vi "OCT Differential.vi"() -> ()   [LabVIEW 2014]
doc: "I. Description:\nThis example demonstrates how to acquire a continuous amount of data (Waveform) using the DAQ device's internal clock.\n\nII. Instructions for Running:\n1. Create an analog input voltage channel.\n2. Set the rate for the sample clock. Additionally, define the sample mode to be continuous.\n3. Call the Start VI to start the acquisition.\n4. Read the waveform data in a loop until the user hits the stop button or an error occurs.\nNote: This example reads data from one or more channels and returns an array of data. Use the Index Array function to access an individual channel of data.\n5. Call the Clear Task VI to clear the Task.\n6. Use the popup dialog box to display an error if any.\n\nIV. I/O Connections Overview:\nMake sure your signal input terminal matches the Physical Channel I/O Control. For further connection information, refer to your hardware reference manual."
uses:
  ATS-VI/ATS_ctl/Device_Ctrl.ctl
  ATS-VI/ATS_ctl/ATS_Async_Ctrl.ctl
  ATS-VI/ATS_ctl/ATS_Async_Mode.ctl
  ATS-VI/ATS_ctl/ATS_DMA_Channel.ctl
  ATS-VI/ATS_ctl/ATS_ReadSamples.ctl
  ATS-VI/ATS_ctl/ATS_Check_Ctrl.ctl
  ATS-VI/ATS_ctl/ClockSource.ctl
  Galvo VIs/galvo_states.ctl
  Signal Processing/processing_states.ctl
  En Face/En Face States.ctl
  Saving Data/Saving Data States.ctl
  Type Defs/OCT Hardware States.ctl
  ATS-VI/ATS_ctl/Range.ctl
  ATS-VI/ATS_ctl/Impedance.ctl
  Type Defs/OCT Imaging Parameters Cluster.ctl
  Classes/Galvo/Scanning Cluster.ctl
  Classes/Galvo/Galvo.lvclass
  Type Defs/OCT DAQ Channel Data Type.ctl
  Type Defs/Display States.ctl
  ATS-VI/ATS_ctl/Coupling.ctl
  ATS-VI/ATS_ctl/Bandwidth.ctl
  ATS-VI/ATS_ctl/InputCtrl.ctl
  ATS-VI/ATS_ctl/TriggerEngine.ctl
  ATS-VI/ATS_ctl/ExtTrigRange.ctl
  ATS-VI/ATS_ctl/ExtTrigger.ctl
  ATS-VI/ATS_ctl/TriggerOperation.ctl
  ATS-VI/ATS_ctl/Trigger.ctl
  ATS-VI/ATS_ctl/ClockRate.ctl
  ATS-VI/ATS_ctl/ClockEdge.ctl
  ATS-VI/ATS_ctl/Clock.ctl
  ATS-VI/ATS_ctl/Record.ctl
  ATS-VI/ATS_ctl/ATS_Global.ctl
  ATS-VI/ATS_ctl/ATS_Async_Status.ctl
  En Face/En Face Depth Parameters.ctl
  ATS-VI/ATS_ctl/ATS_Async_Setting.ctl
panel:
  out "size(s)":i32
  out "First Time?":bool
  out "Save Data":bool
  in  "Async_Setting":T1
  out "Processing Finished":bool
  in  "Imaging Parameters":T2={"Points Per A-Scan"=0, "A-Scans per B-Scan"=0, "Voltage Range"=4.0, "Card Resolution (bits)"=16}
  in  "OCT Hardware States":T3=enum."Save Sweep"
  out "Save State":T4=enum."Initialize"
  out "Clock Length":u32=6304
  out "Reset DAQ":bool
  in  "Tab Control":T5(tab)
  in  "B-Scans Per Buffer":i32=4
  out "Async_Status":T6
  out "Current State":T3=enum."Set Resampling Array"
  in  "Channels":tag="Dev1/ao0:1"
  in  "Trigger Source":tag="/Dev1/PFI7"
  in  "Setup_In":T7={"Record"={"Count"=1, "Presize"=0, "Length"=640}, "Clock"={"ClckSource"=enum."External", "ClckRate"=18, "ClckEdge"=0, "Decimation"=0}, "Input A"={"Coupling"=enum."AC", "Range"=11, "Impedance"=enum."50 ohms", "Bandwidth"=enum."Full Bandwidth"}, "Input B"={"Coupling"=enum."AC", "Range"=4, "Impedance"=enum."50 ohms", "Bandwidth"=enum."Full Bandwidth"}, "Trigger"={"TrigOperation"=enum."Only X", "Timeout (s)"=1.0, "Trig. Delay"=0, "Engine X"={"Source"=enum."External", "Slope"=enum."Positive", "Level"=180}, "Engine Y"={"Source"=enum."Disable", "Slope"=enum."Positive", "Level"=128}, "ExtTrigControl"={"Coupling"=enum."DC", "Range"=enum."5 V"}}} {"Clock"."ClckEdge" items=["Rising", "Falling"]; "Clock"."ClckRate" items=["1 kS/s", "2 kS/s", "5 kS/s", "10 kS/s", "20 kS/s", "50 kS/s", "100 kS/s", "200 kS/s", "500 kS/s", "1 MS/s", "2 MS/s", "5 MS/s", "10 MS/s", "20 MS/s", "25 MS/s", "50 MS/s", "100 MS/s", "125 MS/s", "200 MS/s", "250 MS/s", "500 MS/s", "1 GS/s"]; "Input B"."Range" items=["20mv", "40mV", "50mV", "80mV", "100mV", "200mV", "400mV", "500mV", "800mV", "1 V", "2 V", "4 V", "5 V", "8 V", "10 V", "20 V"]; "Trigger"."Timeout (s)" format="%.2f"; "Input A"."Range" items=["20mv", "40mV", "50mV", "80mV", "100mV", "200mV", "400mV", "500mV", "800mV", "1 V", "2 V", "4 V", "5 V", "8 V", "10 V", "20 V"]}
  in  "Data Format":T23
  out "Channel A or B Phase (or Channel B Raw)":sgl[][](graph)
  out "Channel A or B Intensity (or Channel A Raw)":sgl[][](graph)
  in  "Display":T24
  out "En Face":dbl[][](graph)
  in  "En Face Parameters":T25={"En Face Start\nDepth"=50, "En Face End\nDepth"=200}
  in  "Save Sweep":bool
  in  "Scanning":T26={"Fast Axis Offset"=300.0, "Slow Axis Offset"=1.0, "Slow Axis Amp"=8.0, "Fast Axis Amp"=8.0, "B-scans (rings)"=1, "A(cluster)/B"=0, "Scan Pattern"=enum."Raster"} {"A(cluster)/B" max=1000 step=1; "B-scans (rings)" max=1000 step=1; "Fast Axis Amp" max=20 format="%#.2f"; "Slow Axis Amp" max=20 format="%#.2f"; "Slow Axis Offset" max=10 format="%#.2f"; "Fast Axis Offset" max=10 format="%#.2f"}
  in  "Stop Button":bool
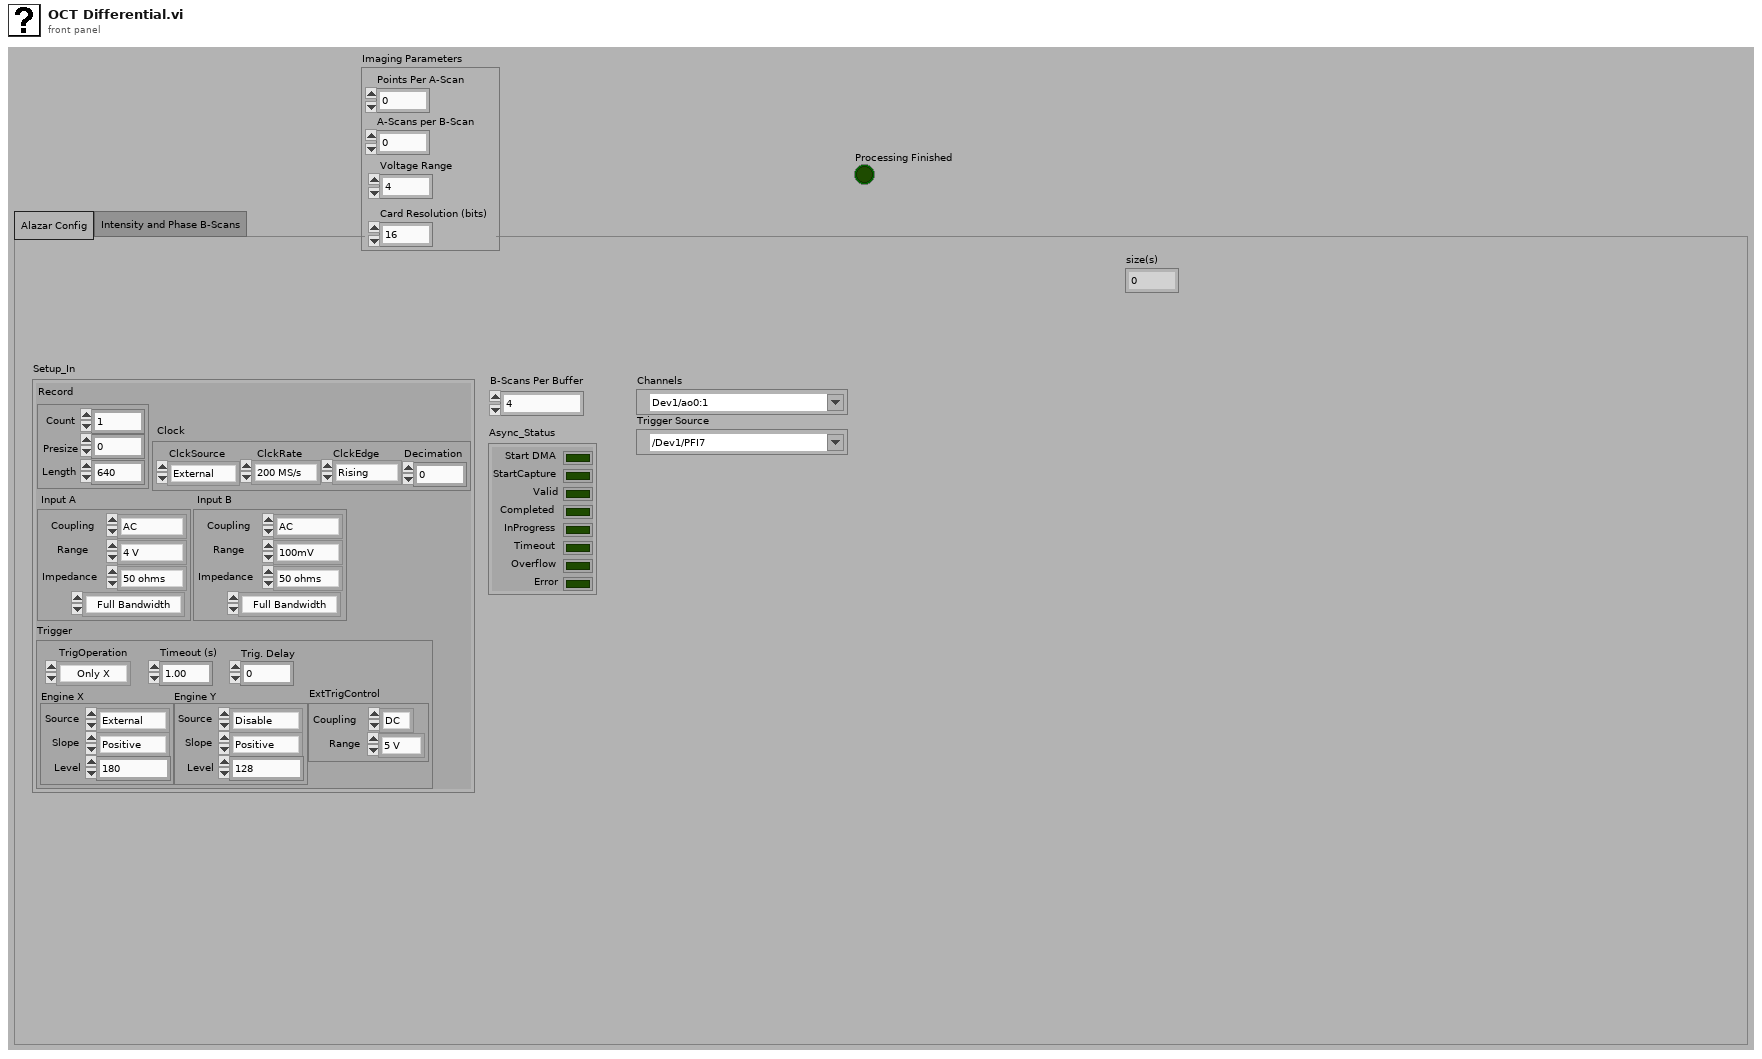
[diagram p1: front panel]
types:
  T1 = typedef "ATS_Async_Setting.ctl" = cluster{"UseHeader":u32, "Rec/Buffer":u32, "Total_Rec":u32, "DataBuffer":bool, "GetProcessedData":bool}
  T2 = typedef "OCT Imaging Parameters Cluster.ctl" = cluster{"Points Per A-Scan":i32, "A-Scans per B-Scan":i32, "Voltage Range":sgl, "Card Resolution (bits)":u16}
  T3 = typedef "OCT Hardware States.ctl" = enum16{"Acquire Data", "Initialize Laser", "Initialize Galvos", "Startup", "Reset DAQ", "Background Subtraction", "Acquire Background", "Update DAQ Parameters", "Stop", "Set Clock", "Initialize DAQ", "Set Resampling Array", "Save Sweep", "Configure Laser"}
  T4 = typedef "Saving Data States.ctl" = enum16{"Get Queue Size", "Get Queue", "Get Timeout", "Flush Queue", "Close Files", "Create Files", "Do Nothing", "Initialize", "Enqueue Data", "Save Data", "Shutdown"}
  T5 = enum32{"Alazar Config", "Intensity and Phase B-Scans"}
  T6 = typedef "ATS_Async_Status.ctl" = cluster{"Start DMA":bool, "StartCapture":bool, "Valid":bool, "Completed":bool, "InProgress":bool, "Timeout":bool, "Overflow":bool, "Error":bool}
  T7 = typedef "ATS_Global.ctl" = cluster{"Record":T8, "Clock":T9, "Input A":T13, "Input B":T13, "Trigger":T18}
  T8 = typedef "Record.ctl" = cluster{"Count":u32, "Presize":u32, "Length":u32}
  T9 = typedef "Clock.ctl" = cluster{"ClckSource":T10, "ClckRate":T11, "ClckEdge":T12, "Decimation":u32}
  T10 = typedef "ClockSource.ctl" = enum16{"Internal", "External", "Medium Ext.", "Slow Ext.", "Ext. AC", "Ext. DC", "Ext. (PLL)"}
  T11 = typedef "ClockRate.ctl" = u32
  T12 = typedef "ClockEdge.ctl" = u16
  T13 = typedef "InputCtrl.ctl" = cluster{"Coupling":T14, "Range":T15, "Impedance":T16, "Bandwidth":T17}
  T14 = typedef "Coupling.ctl" = enum16{"AC", "DC"}
  T15 = typedef "Range.ctl" = u32
  T16 = typedef "Impedance.ctl" = enum16{"1M ohms", "50 ohms"}
  T17 = typedef "Bandwidth.ctl" = enum16{"Full Bandwidth", "Reduce Bandwidth"}
  T18 = typedef "Trigger.ctl" = cluster{"TrigOperation":T19, "Timeout (s)":dbl, "Trig. Delay":u32, "Engine X":T20, "Engine Y":T20, "ExtTrigControl":T21}
  T19 = typedef "TriggerOperation.ctl" = enum16{"Only X", "Only Y", "X or Y", "X and Y", "X xor Y", "X and not Y", "not X and Y"}
  T20 = typedef "TriggerEngine.ctl" = cluster{"Source":enum32{"Chan_A", "Chan_B", "External", "Disable"}, "Slope":enum32{"Positive", "Negative"}, "Level":u32}
  T21 = typedef "ExtTrigger.ctl" = cluster{"Coupling":T14, "Range":T22}
  T22 = typedef "ExtTrigRange.ctl" = enum16{"1 V", "5 V", "TTL"}
  T23 = typedef "OCT DAQ Channel Data Type.ctl" = enum16{"Channel 1", "Channel 2", "Channel 1 and 2"}
  T24 = typedef "Display States.ctl" = enum16{"Channel A", "Channel B"}
  T25 = typedef "En Face Depth Parameters.ctl" = cluster{"En Face Start\nDepth":i32, "En Face End\nDepth":i32}
  T26 = typedef "Galvo.lvclass/Scanning Cluster.ctl" = cluster{"Fast Axis Offset":sgl, "Slow Axis Offset":sgl, "Slow Axis Amp":sgl, "Fast Axis Amp":sgl, "B-scans (rings)":u32, "A(cluster)/B":u32, "Scan Pattern":enum16{"Raster"}}
  T27 = typedef "galvo_states.ctl" = enum16{"Reset", "Reset Galvos?", "Center Galvos", "Register Callback", "Get Scan Parameters", "Show", "Initialize", "Run Raster", "Load Raster", "Run Circle", "Shutdown"}
  T28 = typedef "processing_states.ctl" = enum16{"Initialize", "Set Background", "Update Imaging Parameters", "Get Queue", "Process Data", "Get Size", "Flush Data", "Set Reample Array", "Get Last Processed BScan", "Shutdown"}
  T29 = typedef "Raw Data A and B.ctl" = cluster{"Raw B-Scan Channel A":u16[][][], "Raw B-Scan Channel B":u16[][][]}
  T30 = typedef "Processed OCT Data.ctl" = cluster{"Intensity A":sgl[][][], "Phase A":sgl[][][], "Intensity B":sgl[][][], "Phase B":sgl[][][]}
  T31 = typedef "En Face States.ctl" = enum16{"Save BMP", "Show", "Clear En Face", "Update EnFace"}
  T32 = typedef "ATS_Async_Ctrl.ctl" = enum16{"SetupDMA", "StartCapture", "Get", "Get_Stream", "Abort", "Stop"}
  T33 = typedef "ATS_ReadSamples.ctl" = cluster{"Offset":i32, "Length":u32}
  T34 = typedef "ATS_DMA_Channel.ctl" = enum16{"Channel_A", "Channel_B", "A & B"}
  T35 = typedef "ATS_Async_Mode.ctl" = enum16{"Continuous", "Triggered", "No-Pre-Trigger", "Traditional"}
  T36 = enum16{"No Frequency Enhancement", "Doubled Frequency", "Quadrupled Frequency"}
  T37 = cluster{"low cuttoff":dbl, "high cutoff":dbl, "trimmed length":i32, "front-end samples":i32, "duty cycle (fract)":sgl, "Gage output channel":i32}
  T38 = typedef "ATS_Check_Ctrl.ctl" = enum16{"None", "NO_ATS9462", "ATS9462_Traditional", "Verify Board", "OnBoard Memory", "Board & Memory", "Master/Slave", "NO Master/Slave"}
  T39 = typedef "Device_Ctrl.ctl" = enum16{"Status", "About", "Arm", "ForceTrig", "Abort", "Initialize", "Init (NoPreset)", "Info", "Close", "Calibrate", "SetManually", "LED_ON", "LED_OFF"}
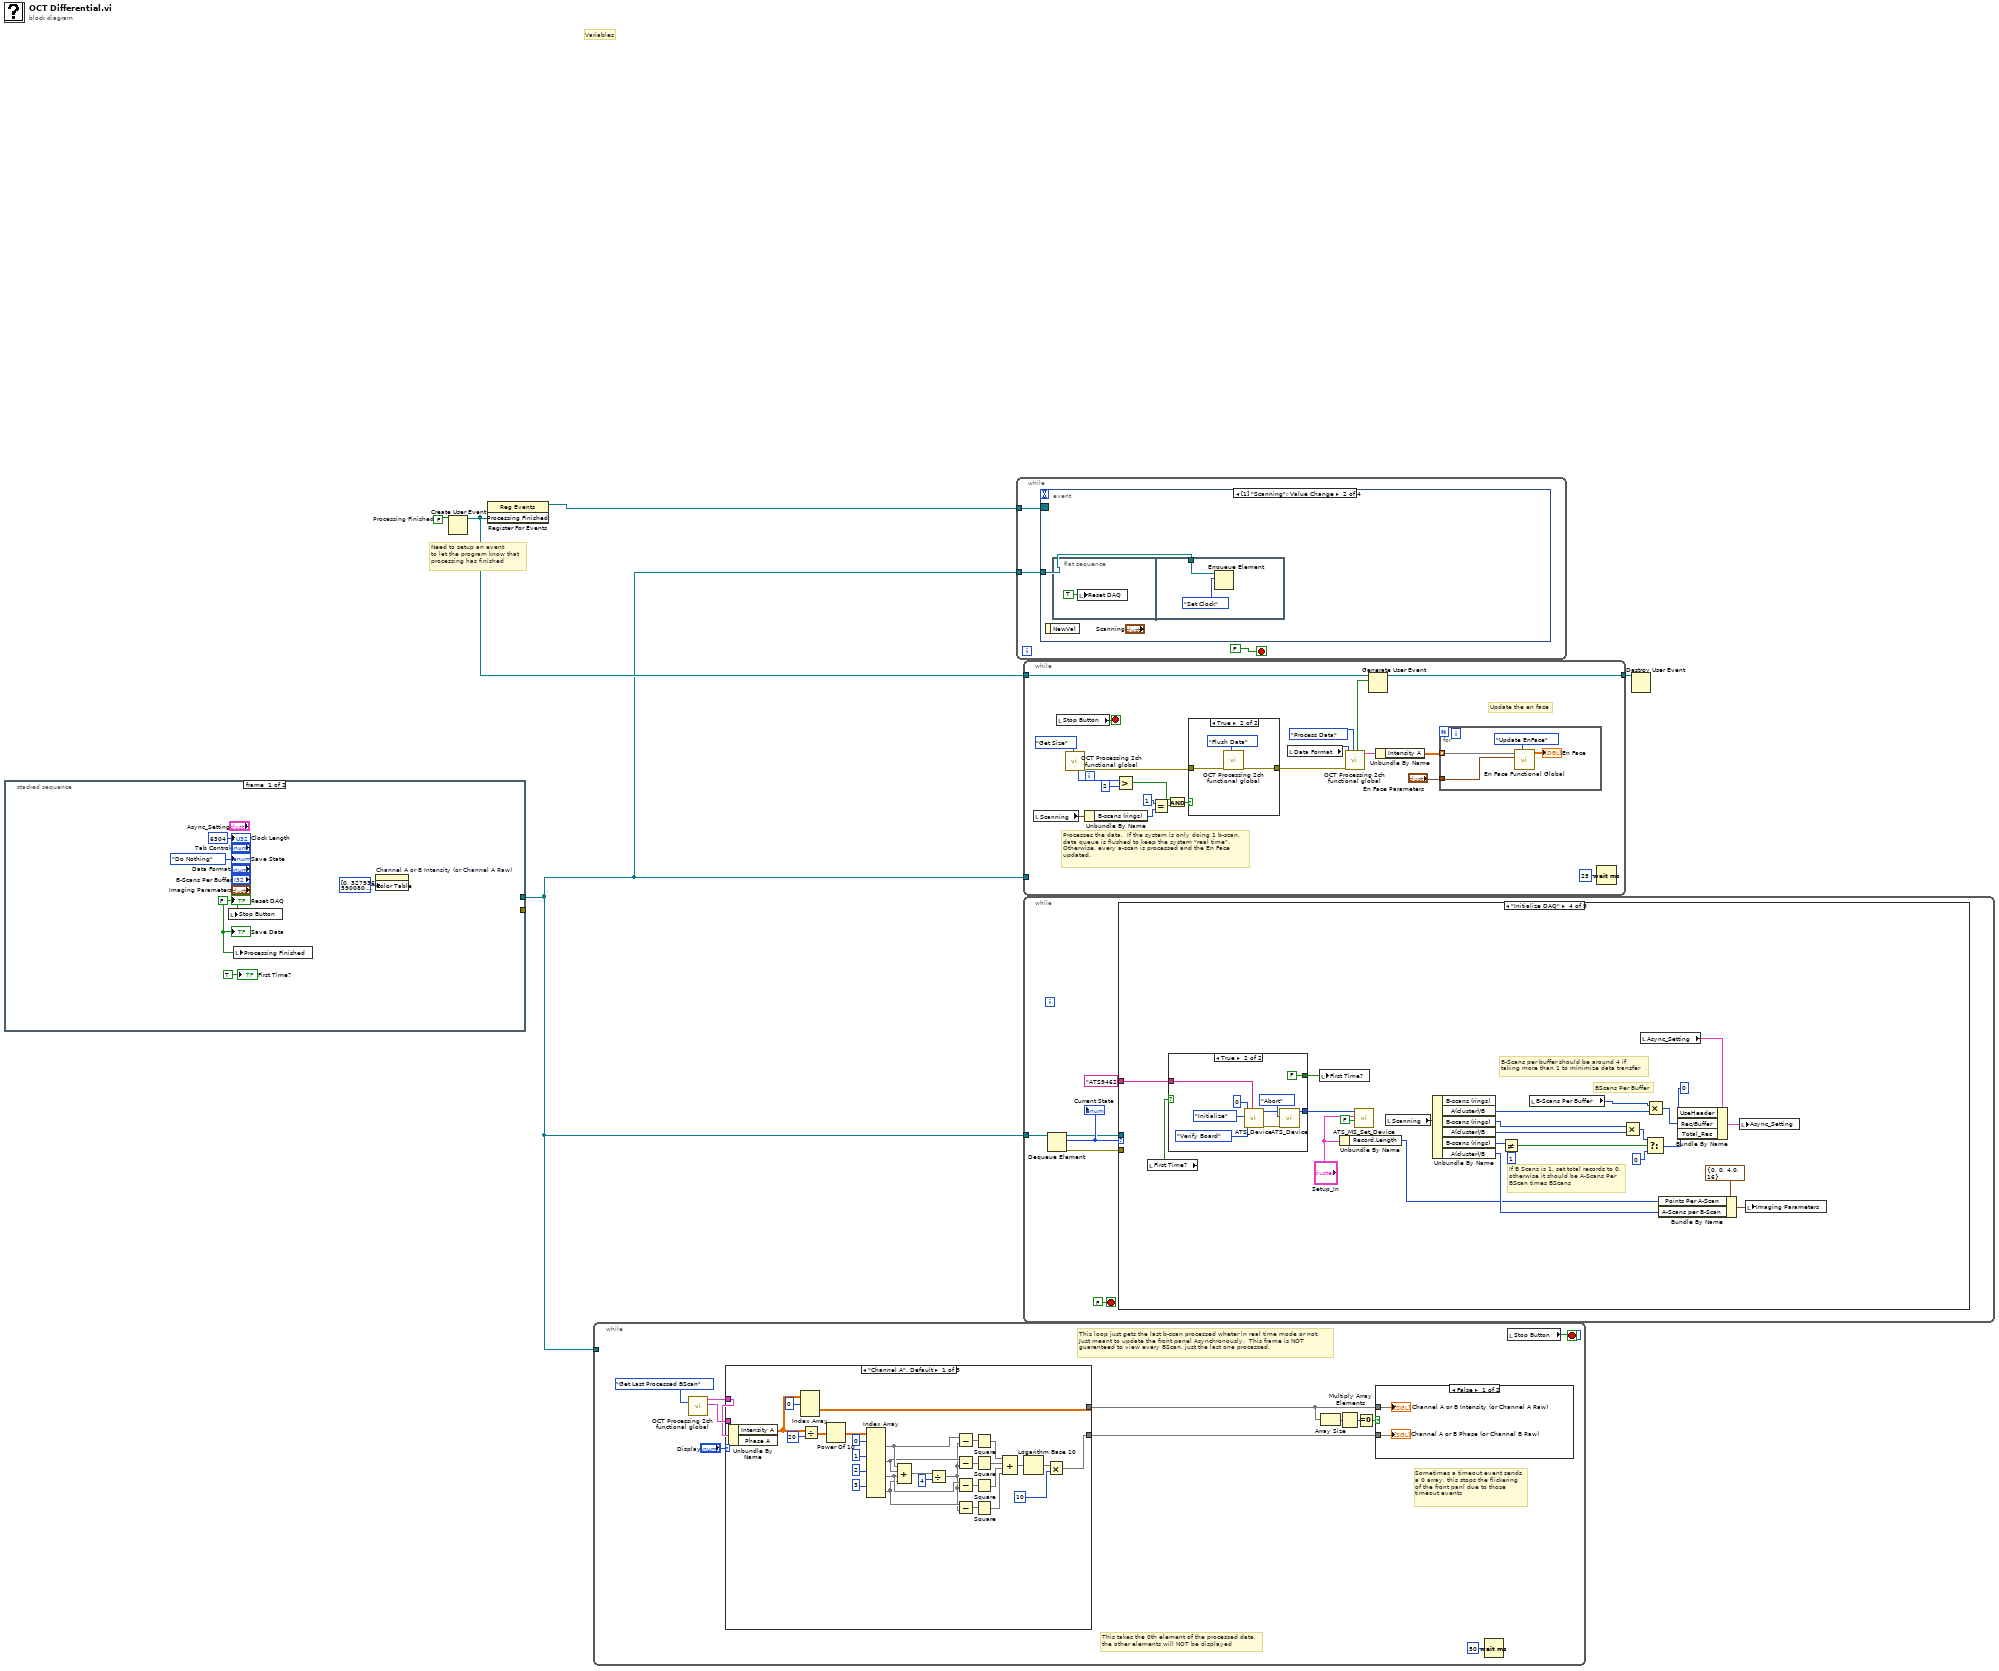
[diagram p0: block diagram]
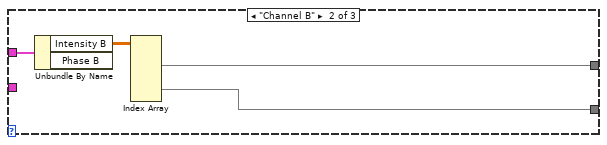
[diagram p4: hidden frame]
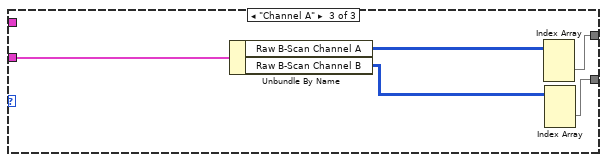
[diagram p5: hidden frame]
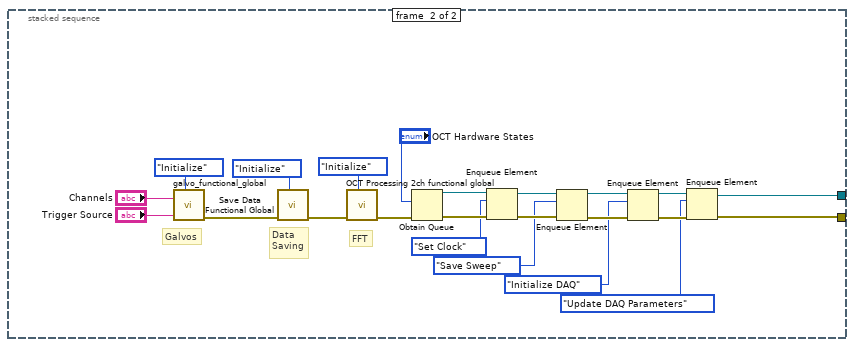
[diagram p6: hidden frame]
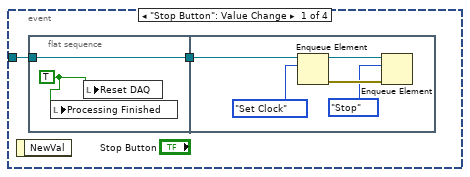
[diagram p7: hidden frame]
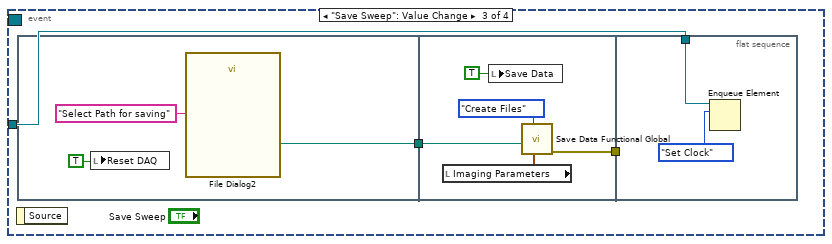
[diagram p8: hidden frame]
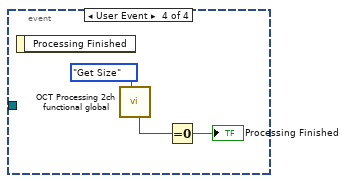
[diagram p9: hidden frame]
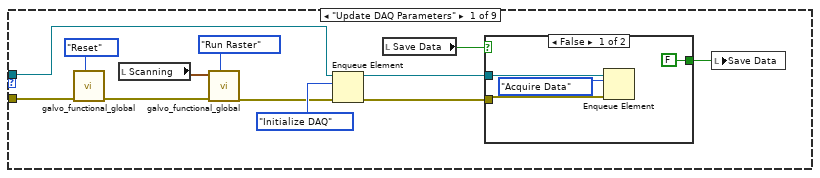
[diagram p10: hidden frame]
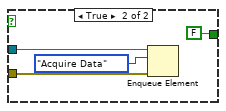
[diagram p11: hidden frame]
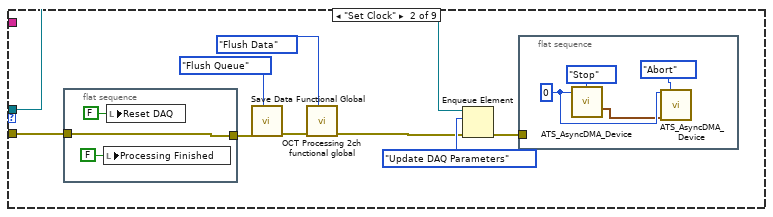
[diagram p12: hidden frame]
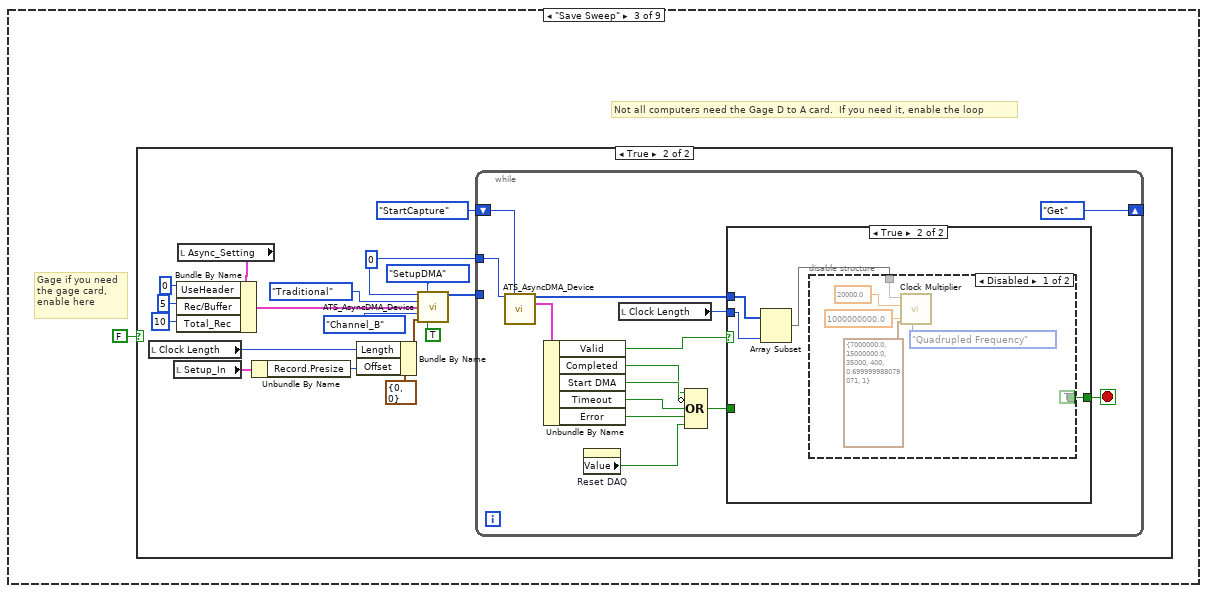
[diagram p13: hidden frame]
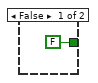
[diagram p17: hidden frame]
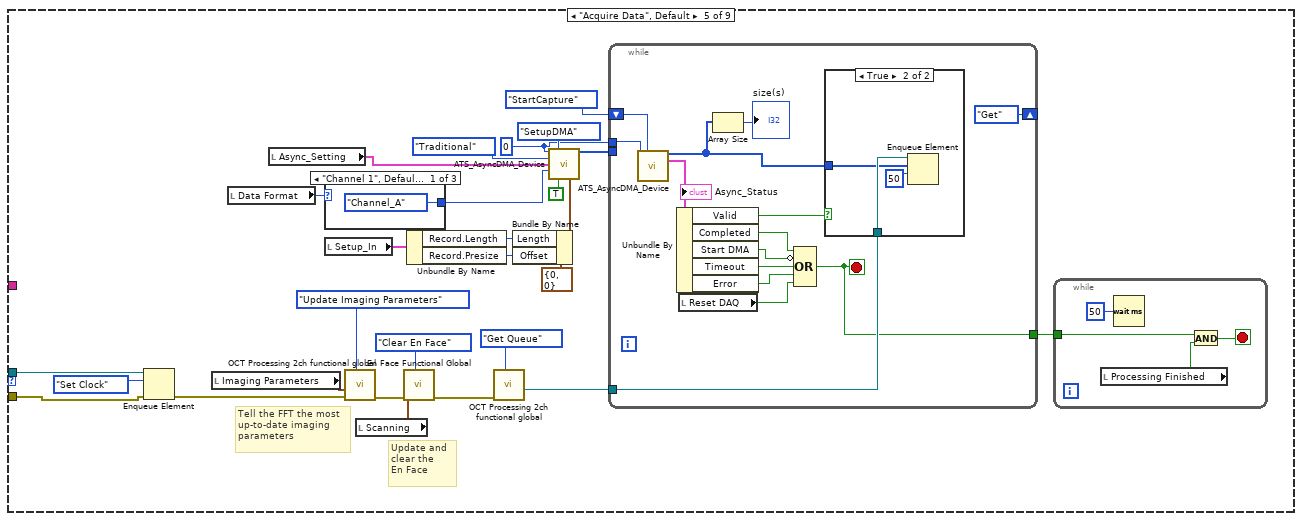
[diagram p18: hidden frame]
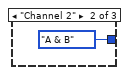
[diagram p19: hidden frame]
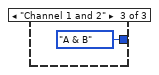
[diagram p20: hidden frame]
diagram:
  w5 = FALSE  # Processing Finished
  # "Need to setup an event \nto let the program know that\nprocessing has finished"
  # "Variables"
  n1 = stacked-sequence {
    tunnel: [_ w19] -> _
    tunnel: [_ w25] -> w1
    frame #0 {
      w7 = FALSE ("Sweep Ready for saving")
      n2 = local write "Stop Button"(w7) -> ()
      n3 = local write "Processing Finished"(w7) -> ()
      n4 = property on="Channel A or B Intensity (or Channel A Raw)" class="IntGraph (strict)"("Color Table"=u32[] [0, 327936, 590080, 852224, 983296, 1114624, 1180160, 1311232, 1442304, 1573632, 1704704, 1770240, 1901312, 1966848, 2098176, 2163712, 2294784, 2491392, 2557184, 2688256, 2753792, 2884864, 2950656, 3081728, 3147264, 3344129, 3475457, 3540993, 3672321, 3738113, 3869185, 3934977, 4066305, 4197633, 4328961, 4394497, 4460289, 4591617, 4657409, 4788481, 4854273, 4985601, 5116929, 5248257, 5314049, 5379841, 5511169, 5576961, 5708033, 5773825, 5905153, 6036482, 6167810, 6233346, 6299138, 6430466, 6496258, 6562050, 6693634, 6759426, 6890754, 7022082, 7087874, 7153666, 7284994, 7350786, 7482114, 7547906, 7613698, 7745026, 7876354, 8007682, 8073474, 8139522, 8205314, 8336642, 8467970, 8533763, 8599555, 8665347, 8731139, 8862467, 8993795, 9059587, 9125380, 9191428, 9257220, 9388548, 9454340, 9520132, 9585924, 9717253, 9848837, 9914629, 9980165, 10045957, 10177541, 10243334, 10309126, 10375174, 10440966, 10572294, 10703623, 10769416, 10835208, 10901256, 10967049, 11033097, 11033609, 11099401, 11165450, 11231242, 11231754, 11297547, 11363339, 11429131, 11495180, 11495692, 11561740, 11693069, 11758861, 11759373, 11825165, 11891214, 11957006, 12022799, 12023311, 12089103, 12220944, 12286736, 12286736, 12352529, 12418577, 12484370, 12550162, 12615954, 12681747, 12747796, 12813588, 12813845, 12879894, 12945686, 13077015, 13142808, 13143064, 13208856, 13274905, 13340697, 13340953, 13472282, 13538075, 13604379, 13670172, 13735964, 13801757, 13867550, 13933343, 13999392, 13999648, 14065441, 14131234, 14197027, 14197541, 14263334, 14329383, 14395176, 14460969, 14592553, 14658346, 14724139, 14789932, 14790189, 14856238, 14922287, 14988080, 15053873, 15054130, 15119923, 15185972, 15251765, 15317559, 15383353, 15449146, 15449660, 15515454, 15515968, 15516226, 15582021, 15582278, 15582536, 15648587, 15648844, 15714639, 15714897, 15715155, 15780949, 15781463, 15847256, 15847770, 15848028, 15913823, 15914081, 15979875, 15980133, 15980391, 16046441, 16046444, 16046703, 16046705, 16112500, 16113015, 16113274, 16113277, 16179072, 16179330, 16179588, 16245384, 16245387, 16245389, 16245648, 16311443, 16376982, 16377241, 16377499, 16443294, 16443553, 16443555, 16443815, 16509866, 16510124, 16510127, 16575923, 16575924, 16576182, 16576441, 16576443, 16576702, 16576705, 16576963, 16577222, 16577224, 16577482, 16577485, 16577743, 16577745, 16578004, 16578262, 16578264, 16578523, 16578782, 16579040, 16579299, 16579301, 16579303, 16579562, 16579821]) -> ()  [unwired: 2 in, 2 out]
      "Clock Length" <- u32 6304 ("Clock Length")
      "Save State" <- Saving_Data_States."Do Nothing" ("Save State")
      "Reset DAQ" <- w7
      "Save Data" <- w7
      "First Time?" <- TRUE ("First Time?")
    }
    frame #1 {
      # "FFT"
      # "Data \nSaving"
      # "Galvos"
      n5 = call "galvo_functional_global.vi"("State"=galvo_states."Initialize", "Trigger Source"="Trigger Source", "Analog Output"="Channels") -> ("error out"=w14:errorcluster)  [unwired: 7 in, 1 out]
      n6 = call "Save Data Functional Global.vi"("States"=Saving_Data_States."Initialize", "error in (no error)"=w14) -> ("error out"=w21:errorcluster)  [unwired: 6 in, 3 out]
      n7 = call "OCT Processing 2ch functional global.vi"("State"=processing_states."Initialize", "error in (no error)"=w21) -> ("error out"=w22:errorcluster)  [unwired: 4 in, 5 out]
      n8 = Obtain Queue(element data type="OCT Hardware States", error in (no error)=w22) -> (queue out=w33:refnum<queue>, error out=w32:errorcluster)  [unwired: 3 in, 1 out]
      n9 = Enqueue Element(queue=w33, element=OCT_Hardware_States."Set Clock", error in (no error)=w32) -> (queue out=w31:refnum<queue>, error out=w30:errorcluster)  [unwired: 1 in, 1 out]
      n10 = Enqueue Element(queue=w31, element=OCT_Hardware_States."Save Sweep", error in (no error)=w30) -> (queue out=w29:refnum<queue>, error out=w28:errorcluster)  [unwired: 1 in, 1 out]
      n11 = Enqueue Element(queue=w29, element=OCT_Hardware_States."Initialize DAQ", error in (no error)=w28) -> (queue out=w27:refnum<queue>, error out=w26:errorcluster)  [unwired: 1 in, 1 out]
      n12 = Enqueue Element(queue=w27, element=OCT_Hardware_States."Update DAQ Parameters", error in (no error)=w26) -> (queue out=w25:refnum<queue>, error out=w19:errorcluster)  [unwired: 1 in, 1 out]
    }
  }
  n13 = Create User Event(user event datatype=w5) -> (user event=w3:refnum<user-event>)  [unwired: 1 in, 1 out]
  n14 = register-events(w3) -> (reference out=w4:refnum<event-registration>)  [unwired: 2 in, 1 out]
  n15 = while {
    tunnel: w1 -> [_]
    stop <- w44 stop-if-true
    # "Sometimes a timeout event sends\na 0 array, this stops the flickering\nof the front panl due to those \ntimeout events"
    # "This takes the 0th element of the processed data,\nthe other elements will NOT be displayed"
    # "This loop just gets the last b-scan processed wheter in real time mode or not. \nJust meant to update the front panel Asynchronously.  This frame is NOT\nguarenteed to view every BScan, just the last one processed."
    n16 = call "OCT Processing 2ch functional global.vi"("State"=processing_states."Get Last Processed BScan") -> ("Raw Data Channel A and B"=w40:T29, "Processed OCT Data"=w38:T30)  [unwired: 5 in, 4 out]
    n17 = case shown="\"Channel A\", Default" "Display" {
      tunnel: w38 -> [w76 w79 _]
      tunnel: w40 -> [_ _ w85]
      tunnel: [w72 w78 w83] -> w36
      tunnel: [w48 w77 w82] -> w39
      frame "Channel A", Default {
        n18 = Unbundle By Name(w76) -> ("Intensity A"=w70:sgl[][][])  [unwired: 1 out]
        n19 = Index Array(array=w70, index (dim 0)=0 ("index (page)")) -> (element=w72:sgl[][])  [unwired: 2 in]
        n20 = Divide(x=w70, y=20) -> (x/y=w71:sgl[][][])
        n21 = Power Of 10(x=w71) -> (10^x=w68:sgl[][][])
        n22 = Index Array(array=w68, index (dim 0) #1=0 ("index (page)"), index (dim 0) #2=1 ("index (page)"), index (dim 0) #3=2 ("index (page)"), index (dim 0) #4=3 ("index (page)")) -> (element #1=w63:sgl[][], element #2=w62:sgl[][], element #3=w61:sgl[][], element #4=w60:sgl[][])  [unwired: 8 in]
        n23 = Compound Arithmetic op=ADD(w63, w62, w61, w60) -> (w74:sgl[][])
        n24 = Divide(x=w74, y=4) -> (x/y=w59:sgl[][])
        n25 = Subtract(x=w63, y=w59) -> (x-y=w58:sgl[][])
        n26 = Subtract(x=w62, y=w59) -> (x-y=w57:sgl[][])
        n27 = Subtract(x=w61, y=w59) -> (x-y=w56:sgl[][])
        n28 = Subtract(x=w60, y=w59) -> (x-y=w55:sgl[][])
        n29 = Square(x=w58) -> (x^2=w54:sgl[][])
        n30 = Square(x=w57) -> (x^2=w53:sgl[][])
        n31 = Square(x=w56) -> (x^2=w52:sgl[][])
        n32 = Square(x=w55) -> (x^2=w51:sgl[][])
        n33 = Compound Arithmetic op=ADD(w54, w53, w52, w51) -> (w50:sgl[][])
        n34 = Logarithm Base 10(1:w50) -> (0:w49:sgl[][])
        n35 = Multiply(x=w49, y=10) -> (x*y=w48:sgl[][])
      }
      frame "Channel B" {
        n36 = Unbundle By Name(w79) -> ("Intensity B"=w80:sgl[][][])  [unwired: 1 out]
        n37 = Index Array(array=w80) -> (element #1=w78:sgl[][], element #2=w77:sgl[][])  [unwired: 6 in]
      }
      frame "Channel A" {
        n38 = Unbundle By Name(w85) -> ("Raw B-Scan Channel A"=w81:u16[][][], "Raw B-Scan Channel B"=w84:u16[][][])
        n39 = Index Array(array=w81) -> (element=w83:u16[][])  [unwired: 3 in]
        n40 = Index Array(array=w84) -> (element=w82:u16[][])  [unwired: 3 in]
      }
    }
    n41 = Array Size(array=w36) -> (size(s)=w37:i32[])
    n42 = Multiply Array Elements(1:w37) -> (0:w35:i32)
    n43 = Equal To 0?(x=w35) -> (x = 0?=w34:bool)
    n44 = case shown="False" w34 {
      tunnel: w39 -> [w46 _]
      tunnel: w36 -> [w45 _]
      frame False {
        "Channel A or B Phase (or Channel B Raw)" <- w46
        "Channel A or B Intensity (or Channel A Raw)" <- w45
      }
      frame True {
      }
    }
    n45 = Wait (ms)(milliseconds to wait=u32 50) -> ()  [unwired: 1 out]
    n46 = local read "Stop Button"() -> (w44:bool)
  }
  n47 = while {
    tunnel: w1 -> [w86]
    tunnel: w4 -> [w87]
    stop <- FALSE stop-if-true
    n48 = event shown="[1] \"Scanning\": Value Change" {
      selector: w87 -> [_ _ _ _]
      dyn-events: _ -> [_ _ _ _]
      timeout: _ -> [_ _ _ _]
      tunnel: w86 -> [w89 w98 w104 _]
      event "Stop Button": Value Change {
        n49 = event-data() -> ()  [unwired: 1 in, 1 out]
        n50 = flat-sequence {
          tunnel: w89 -> [w92]
          tunnel: [w92] -> w90
          tunnel: w90 -> [w97]
          frame #0 {
            w91 = TRUE ("Reset DAQ")
            n51 = local write "Processing Finished"(w91) -> ()
            n52 = local write "Reset DAQ"(w91) -> ()
          }
          frame #1 {
            n53 = Enqueue Element(queue=w97, element=OCT_Hardware_States."Set Clock") -> (queue out=w94:refnum<queue>, error out=w95:errorcluster)  [unwired: 2 in, 1 out]
            n54 = Enqueue Element(queue=w94, element=OCT_Hardware_States."Stop", error in (no error)=w95) -> ()  [unwired: 1 in, 3 out]
          }
        }
      }
      event Value Change {
        n55 = event-data() -> ()  [unwired: 1 in, 1 out]
        n56 = flat-sequence {
          tunnel: w98 -> [w100]
          frame #0 {
            n57 = local write "Reset DAQ"(TRUE ("Reset DAQ")) -> ()
          }
          frame #1 {
            n58 = Enqueue Element(queue=w100, element=OCT_Hardware_States."Set Clock") -> ()  [unwired: 2 in, 3 out]
          }
        }
      }
      event "Save Sweep": Value Change {
        n59 = event-data() -> ()  [unwired: 1 in, 1 out]
        n60 = flat-sequence {
          tunnel: [w105] -> w103
          tunnel: w103 -> [w112]
          tunnel: [w110] -> w102
          tunnel: w104 -> [w114]
          tunnel: w102 -> [_]
          frame #0 {
            n61 = local write "Reset DAQ"(TRUE ("Reset DAQ")) -> ()
            n62 = call "File Dialog2"("prompt"="Select Path for saving") -> ("selected path"=w105:path)  [unwired: 11 in, 3 out]
          }
          frame #1 {
            n63 = local read "Imaging Parameters"() -> (w109:T2)
            n64 = local write "Save Data"(TRUE ("Save Data")) -> ()
            n65 = call "Save Data Functional Global.vi"("Input Parameters"=w109, "States"=Saving_Data_States."Create Files", "Folder"=w112) -> ("error out"=w110:errorcluster)  [unwired: 5 in, 3 out]
          }
          frame #2 {
            n66 = Enqueue Element(queue=w114, element=OCT_Hardware_States."Set Clock") -> ()  [unwired: 2 in, 3 out]
          }
        }
      }
      event User Event {
        n67 = event-data() -> ()  [unwired: 1 in, 1 out]
        n68 = call "OCT Processing 2ch functional global.vi"("State"=processing_states."Get Size") -> ("# elements in queue"=w116:i32)  [unwired: 5 in, 5 out]
        n69 = Equal To 0?(x=w116) -> (x = 0?=→"Processing Finished":bool)
      }
    }
  }
  n70 = while {
    tunnel: w3 -> [w124]
    tunnel: [w122] -> w2
    tunnel: w1 -> [_]
    stop <- w138 stop-if-true
    # "Update the en face"
    # "Processes the data.  If the system is only doing 1 b-scan, \ndata queue is flushed to keep the system \"real time\".\nOtherwise, every a-scan is processed and the En Face\nupdated."
    n71 = local read "Scanning"() -> (w128:T26)
    n72 = local read "Stop Button"() -> (w138:bool)
    n73 = call "OCT Processing 2ch functional global.vi"("State"=processing_states."Get Size") -> ("error out"=w119:errorcluster, "# elements in queue"=w134:i32)  [unwired: 5 in, 4 out]
    n74 = Unbundle By Name(w128) -> ("B-scans (rings)"=w127:u32)
    n75 = Greater?(x=w134, y=2) -> (0:w135:bool)
    n76 = Equal?(x=u32 1, y=w127) -> (x = y?=w126:bool)
    n77 = And(x=w135, y=w126) -> (x .and. y?=w132:bool)
    n78 = case shown="True" w132 {
      tunnel: w119 -> [w143 w146]
      tunnel: [w143 w145] -> w118
      frame False {
      }
      frame True {
        n79 = call "OCT Processing 2ch functional global.vi"("State"=processing_states."Flush Data", "error in (no error)"=w146) -> ("error out"=w145:errorcluster)  [unwired: 4 in, 5 out]
      }
    }
    n80 = local read "Data Format"() -> (w125:T23)
    n81 = call "OCT Processing 2ch functional global.vi"("State"=processing_states."Process Data", "error in (no error)"=w118, "Data Format"=w125) -> ("Processed OCT Data"=w131:T30, "Time Out"=w123:bool)  [unwired: 3 in, 4 out]
    n82 = Generate User Event(user event=w124, event data cluster=w123) -> (user event out=w122:refnum<user-event>)  [unwired: 2 in, 1 out]
    n83 = Unbundle By Name(w131) -> ("Intensity A"=w120:sgl[][][])
    n84 = for {
      tunnel: "En Face Parameters" -> [w141]
      tunnel: w120 -> [w140] mode=indexing
      n85 = call "En Face Functional Global.vi"(7:En_Face_States."Update EnFace" ("En Face States"), 10:w141, "Intensity Graph 2"=w140) -> ("Intensity Graph"=→"En Face":dbl[][])  [unwired: 7 in, 1 out]
    }
    n86 = Wait (ms)(milliseconds to wait=u32 25) -> ()  [unwired: 1 out]
  }
  n87 = while {
    tunnel: w1 -> [w152]
    stop <- FALSE stop-if-true
    n88 = Dequeue Element(queue=w152) -> (queue out=w148:refnum<queue>, element=w150:T3, error out=w149:errorcluster)  [unwired: 2 in, 1 out]
    "Current State" <- w150
    n89 = case shown="\"Initialize DAQ\"" w150 {
      tunnel: w149 -> [w160 w176 _ _ w270 w319 _ w394 _]
      tunnel: w148 -> [w158 w178 _ _ w279 w336 _ w395 _]
      tunnel: "ATS9462" ("BoardToVerify") -> [_ _ _ w238 _ _ _ _ w401]
      frame "Update DAQ Parameters" {
        n90 = call "galvo_functional_global.vi"("State"=galvo_states."Reset", "error in (no error)"=w160) -> ("error out"=w163:errorcluster)  [unwired: 8 in, 1 out]
        n91 = local read "Scanning"() -> (w161:T26)
        n92 = call "galvo_functional_global.vi"("State"=galvo_states."Run Raster", "error in (no error)"=w163, "user event out"=w161) -> ("error out"=w157:errorcluster)  [unwired: 7 in, 1 out]
        n93 = Enqueue Element(queue=w158, element=OCT_Hardware_States."Initialize DAQ", error in (no error)=w157) -> (queue out=w156:refnum<queue>, error out=w155:errorcluster)  [unwired: 1 in, 1 out]
        n94 = local read "Save Data"() -> (w154:bool)
        n95 = case shown="False" w154 {
          tunnel: w156 -> [w167 w172]
          tunnel: w155 -> [w166 w171]
          tunnel: [FALSE ("Reset DAQ") FALSE ("Reset DAQ")] -> w153
          frame False {
            n96 = Enqueue Element(queue=w167, element=OCT_Hardware_States."Acquire Data", error in (no error)=w166) -> ()  [unwired: 1 in, 3 out]
          }
          frame True {
            n97 = Enqueue Element(queue=w172, element=OCT_Hardware_States."Acquire Data", error in (no error)=w171) -> ()  [unwired: 1 in, 3 out]
          }
        }
        n98 = local write "Save Data"(w153) -> ()
      }
      frame "Set Clock" {
        n99 = flat-sequence {
          tunnel: w176 -> [w187]
          tunnel: [w187] -> w175
          frame #0 {
            n100 = local write "Processing Finished"(FALSE ("Reset DAQ")) -> ()
            n101 = local write "Reset DAQ"(FALSE ("Reset DAQ")) -> ()
          }
        }
        n102 = call "Save Data Functional Global.vi"("States"=Saving_Data_States."Flush Queue", "error in (no error)"=w175) -> ("error out"=w180:errorcluster)  [unwired: 6 in, 3 out]
        n103 = call "OCT Processing 2ch functional global.vi"("State"=processing_states."Flush Data", "error in (no error)"=w180) -> ("error out"=w173:errorcluster)  [unwired: 4 in, 5 out]
        n104 = Enqueue Element(queue=w178, element=OCT_Hardware_States."Update DAQ Parameters", error in (no error)=w173) -> (error out=w174:errorcluster)  [unwired: 1 in, 2 out]
        n105 = flat-sequence {
          tunnel: w174 -> [_]
          frame #0 {
            w185 = 0 ("DeviceIn")
            n106 = call "ATS_AsyncDMA_Device.vi"("DeviceIn"=w185, "ATS_Async_Ctrl"=ATS_Async_Ctrl."Stop") -> ("ReadSamples_Out"=w184:T33)  [unwired: 9 in, 4 out]
            n107 = call "ATS_AsyncDMA_Device.vi"("DeviceIn"=w185, "ATS_Async_Ctrl"=ATS_Async_Ctrl."Abort", "ReadSamples"=w184) -> ()  [unwired: 8 in, 5 out]
          }
        }
      }
      frame "Save Sweep" {
        # "Gage if you need\nthe gage card,\nenable here"
        # "Not all computers need the Gage D to A card.  If you need it, enable the loop"
        n108 = case shown="True" FALSE {
          frame False {
          }
          frame True {
            w192 = 0 ("DeviceIn")
            n109 = local read "Clock Length"() -> (w194:u32)
            n110 = local read "Setup_In"() -> (w196:T7)
            n111 = local read "Async_Setting"() -> (w190:T1)
            n112 = Bundle By Name(cluster=w190, "UseHeader"=u32 0, "Rec/Buffer"=u32 5, "Total_Rec"=u32 10) -> (w191:T1)
            n113 = Unbundle By Name(w196) -> ("Record.Presize"=w195:u32)
            n114 = Bundle By Name(cluster=T33 {"Offset"=0, "Length"=0} ("ReadSamples"), "Length"=w194, "Offset"=w195) -> (w193:T33)
            n115 = call "ATS_AsyncDMA_Device.vi"("DeviceIn"=w192, "ATS_Async_Ctrl"=ATS_Async_Ctrl."SetupDMA" ("ATS_DMA_Ctrl"), "Async_Mode"=ATS_Async_Mode."Traditional", "Async_Setting"=w191, "Channel"=ATS_DMA_Channel."Channel_B", "ReadSamples"=w193, "Start Now / Wait"=TRUE) -> ("Buffer"=w201:u16[])  [unwired: 4 in, 4 out]
            n116 = while {
              tunnel: w201 -> [_]
              shift-right: [ATS_Async_Ctrl."Get" ("ATS_Async_Ctrl")] -> _
              shift-left: ATS_Async_Ctrl."StartCapture" ("ATS_Async_Ctrl") -> [w216]
              tunnel: w192 -> [w207]
              stop <- w211 stop-if-true
              n117 = call "ATS_AsyncDMA_Device.vi"("DeviceIn"=w207, "ATS_Async_Ctrl"=w216) -> ("Buffer"=w209:u16[], "Async_Status"=w214:T6)  [unwired: 9 in, 3 out]
              n118 = Unbundle By Name(w214) -> ("Valid"=w212:bool, "Completed"=w218:bool, "Start DMA"=w219:bool, "Timeout"=w220:bool, "Error"=w217:bool)
              n119 = property on="Reset DAQ" class="Bool (strict)"() -> ("Value"=w213:bool)  [unwired: 2 in, 2 out]
              n120 = local read "Clock Length"() -> (w208:u32)
              n121 = Compound Arithmetic op=OR(w218, invert w219, w220, w217, w213) -> (w210:bool)
              n122 = case shown="True" w212 {
                tunnel: w209 -> [_ w224]
                tunnel: [w221 w225] -> w211
                tunnel: w210 -> [w221 _]
                tunnel: w208 -> [_ w223]
                frame False {
                }
                frame True {
                  n123 = Array Subset(array=w224, length=w223) -> (w222:u16[])  [unwired: 1 in]
                  n124 = disable-structure shown="Disabled" {
                    disable-tunnel: [TRUE _] -> w225
                    disable-tunnel: w222 -> [w230 _]
                    frame Disabled {
                      w227 = 1000000000.0 items=["Slow Gage"=300000000.0, "Fast Gage"=1000000000.0] ("Gage Speed")
                      n125 = call "Clock Multiplier.vi"("Enum"=T36."Quadrupled Frequency", "Clock Gen Params"=T37 {"low cuttoff"=7000000.0, "high cutoff"=15000000.0, "trimmed length"=35000, "front-end samples"=400, "duty cycle (fract)"=0.7, "Gage output channel"=1}, "Gage Speed"=w227, "Sweep Speed"=20000.0, "k-space signal in"=w230) -> ()  [unwired: 6 in, 1 out]
                    }
                    frame Enabled {
                    }
                  }
                }
              }
            }
          }
        }
      }
      frame "Initialize DAQ" {
        # "B-Scans per buffer should be around 4 if \ntaking more than 1 to minimize data transfer"
        # "If B Scans is 1, set total records to 0,\notherwise it should be A-Scans Per\nBScan times BScans"
        # "BScans Per Buffer"
        n126 = local read "First Time?"() -> (w234:bool)
        n127 = case shown="True" w234 {
          tunnel: [_ w262] -> w256
          tunnel: w238 -> [_ w259]
          tunnel: [FALSE ("First Time?") FALSE ("First Time?")] -> w233
          frame False {
          }
          frame True {
            n128 = call "ATS_Device.vi"("BoardToVerify"=w259, "ATS_Check"=ATS_Check_Ctrl."Verify Board", "DevCtrl"=Device_Ctrl."Initialize", "DeviceIn"=0 ("Device")) -> ("error out"=w260:errorcluster, "DeviceOut"=w264:i32)  [unwired: 1 in, 5 out]
            n129 = call "ATS_Device.vi"("error in (no error)"=w260, "DevCtrl"=Device_Ctrl."Abort", "DeviceIn"=w264) -> ("DeviceOut"=w262:i32)  [unwired: 2 in, 6 out]
          }
        }
        n130 = local write "First Time?"(w233) -> ()
        n131 = Unbundle By Name("Setup_In") -> ("Record.Length"=w239:u32)
        n132 = call "ATS_MS_Set_Device.vi"("Set_Manually (F)"=FALSE, "Setup_In"="Setup_In", "DeviceIn"=w256) -> ()  [unwired: 3 in, 6 out]
        n133 = local read "Scanning"() -> (w252:T26)
        n134 = Unbundle By Name(w252) -> ("A(cluster)/B"=w250:u32, "B-scans (rings)"=w249:u32, "A(cluster)/B"=w248:u32, "B-scans (rings)"=w246:u32, "A(cluster)/B"=w241:u32)  [unwired: 1 out]
        n135 = Not Equal?(x=w246, y=u32 1 ("x")) -> (x != y?=w247:bool)
        n136 = local read "B-Scans Per Buffer"() -> (w232:i32)
        n137 = Multiply(x=w249, y=w248) -> (x*y=w244:u32)
        n138 = local read "Async_Setting"() -> (w237:T1)
        n139 = Select(t=w244, s=w247, f=u32 0 ("Total_Rec")) -> (s? t:f=w254:u32)
        n140 = Multiply(x=w232, y=w250) -> (x*y=w251:u32)
        n141 = Bundle By Name(cluster=T2 {"Points Per A-Scan"=0, "A-Scans per B-Scan"=0, "Voltage Range"=4.0, "Card Resolution (bits)"=16} ("Imaging Parameters"), "Points Per A-Scan"=w239, "A-Scans per B-Scan"=w241) -> (w240:T2)
        n142 = Bundle By Name(cluster=w237, "UseHeader"=u32 0, "Rec/Buffer"=w251, "Total_Rec"=w254) -> (w236:T1)
        n143 = local write "Async_Setting"(w236) -> ()
        n144 = local write "Imaging Parameters"(w240) -> ()
      }
      frame "Acquire Data", Default {
        w288 = 0 ("DeviceIn")
        # "Update and \nclear the \nEn Face"
        # "Tell the FFT the most\nup-to-date imaging\nparameters"
        n145 = Enqueue Element(queue=w279, element=OCT_Hardware_States."Set Clock", error in (no error)=w270) -> (error out=w269:errorcluster)  [unwired: 1 in, 2 out]
        n146 = local read "Imaging Parameters"() -> (w276:T2)
        n147 = local read "Data Format"() -> (w281:T23)
        n148 = local read "Async_Setting"() -> (w274:T1)
        n149 = case shown="\"Channel 1\", Default" w281 {
          tunnel: [ATS_DMA_Channel."Channel_A" ("Channel") ATS_DMA_Channel."A & B" ("Channel") ATS_DMA_Channel."A & B" ("Channel")] -> w280
          frame "Channel 1", Default {
          }
          frame "Channel 2" {
          }
          frame "Channel 1 and 2" {
          }
        }
        n150 = local read "Setup_In"() -> (w284:T7)
        n151 = call "OCT Processing 2ch functional global.vi"("State"=processing_states."Update Imaging Parameters", "error in (no error)"=w269, "Input Parameters"=w276) -> ("error out"=w278:errorcluster)  [unwired: 3 in, 5 out]
        n152 = local read "Scanning"() -> (w273:T26)
        n153 = call "En Face Functional Global.vi"(7:En_Face_States."Clear En Face" ("En Face States"), "Error In"=w278, 9:w273) -> ("Error Out"=w272:errorcluster)  [unwired: 7 in, 1 out]
        n154 = Unbundle By Name(w284) -> ("Record.Length"=w283:u32, "Record.Presize"=w282:u32)
        n155 = call "OCT Processing 2ch functional global.vi"("State"=processing_states."Get Queue", "error in (no error)"=w272) -> ("queue out"=w268:refnum<queue>)  [unwired: 4 in, 5 out]
        n156 = Bundle By Name(cluster=T33 {"Offset"=0, "Length"=0} ("ReadSamples"), "Length"=w283, "Offset"=w282) -> (w290:T33)
        n157 = call "ATS_AsyncDMA_Device.vi"("DeviceIn"=w288, "ATS_Async_Ctrl"=ATS_Async_Ctrl."SetupDMA" ("ATS_DMA_Ctrl"), "Async_Mode"=ATS_Async_Mode."Traditional", "Async_Setting"=w274, "Channel"=w280, "ReadSamples"=w290, "Start Now / Wait"=TRUE) -> ("Buffer"=w286:u16[])  [unwired: 4 in, 4 out]
        n158 = while {
          tunnel: w286 -> [_]
          tunnel: w288 -> [w314]
          shift-right: [ATS_Async_Ctrl."Get" ("ATS_Async_Ctrl")] -> _
          shift-left: ATS_Async_Ctrl."StartCapture" ("ATS_Async_Ctrl") -> [w311]
          tunnel: w268 -> [w304]
          tunnel: [w303] -> w267
          stop <- w303 stop-if-true
          n159 = call "ATS_AsyncDMA_Device.vi"("DeviceIn"=w314, "ATS_Async_Ctrl"=w311) -> ("Buffer"=w301:u16[], "Async_Status"=w309:T6)  [unwired: 9 in, 3 out]
          "Async_Status" <- w309
          n160 = Unbundle By Name(w309) -> ("Valid"=w308:bool, "Completed"=w305:bool, "Start DMA"=w306:bool, "Timeout"=w313:bool, "Error"=w312:bool)
          n161 = local read "Reset DAQ"() -> (w307:bool)
          n162 = Array Size(array=w301) -> (size(s)=→"size(s)":i32)
          n163 = Compound Arithmetic op=OR(w305, invert w306, w313, w312, w307) -> (w303:bool)
          n164 = case shown="True" w308 {
            tunnel: w301 -> [_ w316]
            tunnel: w304 -> [_ w317]
            frame False {
              # "Do nothing"
            }
            frame True {
              n165 = Enqueue Element(queue=w317, element=w316, timeout in ms (-1)=50) -> ()  [unwired: 1 in, 3 out]
            }
          }
        }
        n166 = while {
          tunnel: w267 -> [w297]
          stop <- w295 stop-if-true
          n167 = local read "Processing Finished"() -> (w296:bool)
          n168 = Wait (ms)(milliseconds to wait=u32 50) -> ()  [unwired: 1 out]
          n169 = And(x=w297, y=w296) -> (x .and. y?=w295:bool)
        }
      }
      frame "Acquire Data" {
        w345 = 0 ("DeviceIn")
        # "Close files and set save \nstate to do nothing"
        # "Update and \nclear the \nEn Face"
        # "Tell the FFT the most\nup-to-date imaging\nparameters"
        n170 = local read "Imaging Parameters"() -> (w333:T2)
        n171 = local read "Data Format"() -> (w338:T23)
        n172 = local read "Async_Setting"() -> (w327:T1)
        n173 = case shown="\"Channel 1\", Default" w338 {
          tunnel: [ATS_DMA_Channel."Channel_A" ("Channel") ATS_DMA_Channel."A & B" ("Channel") ATS_DMA_Channel."A & B" ("Channel")] -> w337
          frame "Channel 1", Default {
          }
          frame "Channel 2" {
          }
          frame "Channel 1 and 2" {
          }
        }
        n174 = local read "Setup_In"() -> (w341:T7)
        n175 = call "OCT Processing 2ch functional global.vi"("State"=processing_states."Update Imaging Parameters", "error in (no error)"=w319, "Input Parameters"=w333) -> ("error out"=w335:errorcluster)  [unwired: 3 in, 5 out]
        n176 = local read "Scanning"() -> (w326:T26)
        n177 = call "En Face Functional Global.vi"(7:En_Face_States."Clear En Face" ("En Face States"), "Error In"=w335, 9:w326) -> ("Error Out"=w325:errorcluster)  [unwired: 7 in, 1 out]
        n178 = Unbundle By Name(w341) -> ("Record.Length"=w340:u32, "Record.Presize"=w339:u32)
        n179 = call "Save Data Functional Global.vi"("States"=Saving_Data_States."Get Queue", "error in (no error)"=w319) -> ("Saving Queue Out"=w320:refnum<queue>)  [unwired: 6 in, 3 out]
        n180 = call "OCT Processing 2ch functional global.vi"("State"=processing_states."Get Queue", "error in (no error)"=w325) -> ("error out"=w324:errorcluster, "queue out"=w322:refnum<queue>)  [unwired: 4 in, 4 out]
        n181 = Bundle By Name(cluster=T33 {"Offset"=0, "Length"=0} ("ReadSamples"), "Length"=w340, "Offset"=w339) -> (w347:T33)
        n182 = call "ATS_AsyncDMA_Device.vi"("DeviceIn"=w345, "ATS_Async_Ctrl"=ATS_Async_Ctrl."SetupDMA" ("ATS_DMA_Ctrl"), "Async_Mode"=ATS_Async_Mode."Traditional", "Async_Setting"=w327, "Channel"=w337, "ReadSamples"=w347, "Start Now / Wait"=TRUE) -> ("Buffer"=w343:u16[])  [unwired: 4 in, 4 out]
        n183 = while {
          tunnel: w324 -> [_]
          tunnel: [w356] -> w332
          i -> [w355]
          stop <- w354 stop-if-true
          # "Saves data as long as data is being fed into the Queue,\notherwise it will time out and halt this loop."
          n184 = case shown="1, Default" w355 {
            tunnel: [FALSE w362] -> w354
            tunnel: [_ w359] -> w356
            frame 0 {
              # "Wait for data to Q up"
              n185 = Wait (ms)(milliseconds to wait=u32 500) -> ()  [unwired: 1 out]
            }
            frame 1, Default {
              n186 = local read "Data Format"() -> (w365:T23)
              n187 = Wait (ms)(milliseconds to wait=u32 100) -> ()  [unwired: 1 out]
              n188 = call "Save Data Functional Global.vi"("States"=Saving_Data_States."Save Data", "Data Format"=w365) -> ("error out"=w360:errorcluster)  [unwired: 6 in, 3 out]
              n189 = call "Save Data Functional Global.vi"("States"=Saving_Data_States."Get Queue Size", "error in (no error)"=w360) -> ("error out"=w359:errorcluster, "# elements in queue"=w361:i32)  [unwired: 6 in, 2 out]
              n190 = Equal To 0?(x=w361) -> (x = 0?=w362:bool)
            }
          }
        }
        n191 = while {
          tunnel: w343 -> [_]
          tunnel: w345 -> [w380]
          shift-right: [ATS_Async_Ctrl."Get" ("ATS_Async_Ctrl")] -> _
          shift-left: ATS_Async_Ctrl."StartCapture" ("ATS_Async_Ctrl") -> [w377]
          tunnel: w322 -> [w370]
          tunnel: w320 -> [w369]
          stop <- w368 stop-if-true
          n192 = call "ATS_AsyncDMA_Device.vi"("DeviceIn"=w380, "ATS_Async_Ctrl"=w377) -> ("Buffer"=w367:u16[], "Async_Status"=w375:T6)  [unwired: 9 in, 3 out]
          n193 = Unbundle By Name(w375) -> ("Valid"=w374:bool, "Completed"=w371:bool, "Start DMA"=w372:bool, "Timeout"=w379:bool, "Error"=w378:bool)
          n194 = local read "Reset DAQ"() -> (w373:bool)
          n195 = Compound Arithmetic op=OR(w371, invert w372, w379, w378, w373) -> (w368:bool)
          n196 = case shown="True" w374 {
            tunnel: w367 -> [_ w383]
            tunnel: w367 -> [_ w384]
            tunnel: w370 -> [_ w385]
            tunnel: w369 -> [_ w382]
            frame False {
              # "Do nothing"
            }
            frame True {
              w381 = 50 ("timeout in ms (-1)")
              n197 = Enqueue Element(queue=w382, element=w383, timeout in ms (-1)=w381) -> ()  [unwired: 1 in, 3 out]
              n198 = Enqueue Element(queue=w385, element=w384, timeout in ms (-1)=w381) -> ()  [unwired: 1 in, 3 out]
            }
          }
        }
        n199 = call "Save Data Functional Global.vi"("States"=Saving_Data_States."Close Files", "error in (no error)"=w332) -> ("error out"=w331:errorcluster)  [unwired: 6 in, 3 out]
        n200 = call "Save Data Functional Global.vi"("States"=Saving_Data_States."Do Nothing" ("Save State"), "error in (no error)"=w331) -> ("error out"=w329:errorcluster)  [unwired: 6 in, 3 out]
        n201 = Enqueue Element(queue=w336, element=OCT_Hardware_States."Set Clock", error in (no error)=w329) -> ()  [unwired: 1 in, 3 out]
      }
      frame "Set Resampling Array" {
        n202 = Wait (ms)(milliseconds to wait=u32 10) -> ()  [unwired: 1 out]
      }
      frame "Stop" {
        n203 = Release Queue(queue=w395, error in (no error)=w394) -> (error out=w393:errorcluster)  [unwired: 1 in, 2 out]
        n204 = call "OCT Processing 2ch functional global.vi"("State"=processing_states."Shutdown", "error in (no error)"=w393) -> ("error out"=w392:errorcluster)  [unwired: 4 in, 5 out]
        n205 = call "Save Data Functional Global.vi"("States"=Saving_Data_States."Shutdown", "error in (no error)"=w392) -> ("error out"=w389:errorcluster)  [unwired: 6 in, 3 out]
        n206 = call "galvo_functional_global.vi"("State"=galvo_states."Shutdown", "error in (no error)"=w389) -> ("error out"=w388:errorcluster)  [unwired: 8 in, 1 out]
        n207 = flat-sequence {
          tunnel: w388 -> [_]
          frame #0 {
            w399 = 0 ("DeviceIn")
            n208 = call "ATS_AsyncDMA_Device.vi"("DeviceIn"=w399, "ATS_Async_Ctrl"=ATS_Async_Ctrl."Stop") -> ("ReadSamples_Out"=w398:T33)  [unwired: 9 in, 4 out]
            n209 = call "ATS_AsyncDMA_Device.vi"("DeviceIn"=w399, "ATS_Async_Ctrl"=ATS_Async_Ctrl."Abort", "ReadSamples"=w398) -> ()  [unwired: 8 in, 5 out]
          }
          frame #1 {
            n210 = Stop(stop? (T)=TRUE) -> ()
          }
        }
      }
      frame "Set Clock" {
        w403 = T15 12 items=["20mV", "40mV", "50mV", "80mV", "100mV", "200mV", "400mV", "500mV", "800mV", "1 V", "1.25 V", "2 V", "4 V", "5 V", "8 V", "10 V", "16 V", "20 V", "40 V", "HiFi"] ("Input B.Range")
        w407 = u32 18 items=["1 kS/s", "2 kS/s", "5 kS/s", "10 kS/s", "20 kS/s", "50 kS/s", "100 kS/s", "200 kS/s", "500 kS/s", "1 MS/s", "2 MS/s", "5 MS/s", "10 MS/s", "20 MS/s", "50 MS/s", "100 MS/s", "125 MS/s", "160 MS/s", "180 MS/s"] ("ClckRate")
        n211 = local read "Clock Length"() -> (w406:u32)
        n212 = call "ATS_Device.vi"("BoardToVerify"=w401, "ATS_Check"=ATS_Check_Ctrl."Verify Board", "DevCtrl"=Device_Ctrl."Initialize", "DeviceIn"=0 ("Device")) -> ("error out"=w409:errorcluster, "DeviceOut"=w414:i32)  [unwired: 1 in, 5 out]
        n213 = call "ATS_Device.vi"("error in (no error)"=w409, "DevCtrl"=Device_Ctrl."Abort", "DeviceIn"=w414) -> ("DeviceOut"=w412:i32)  [unwired: 2 in, 6 out]
        n214 = local read "Setup_In"() -> (w405:T7)
        n215 = Bundle By Name(cluster=w405, "Record.Length"=w406, "Clock.ClckSource"=ClockSource."Internal", "Clock.ClckRate"=w407, "Input B.Range"=w403, "Input A.Impedance"=Impedance."50 ohms") -> (w404:T7)
        n216 = call "ATS_MS_Set_Device.vi"("Set_Manually (F)"=FALSE, "Setup_In"=w404, "DeviceIn"=w412) -> ()  [unwired: 3 in, 6 out]
      }
    }
  }
  n217 = Destroy User Event(user event=w2) -> ()  [unwired: 1 in, 1 out]
